vi "internalTesting.vi"() -> ()   [LabVIEW 2017, in "LabVIEW NPOI.lvlib" / "MS-Word.lvclass"]
uses:
  MS-Word.lvclass
  C:/Users/Neo/Desktop/Dev_Tools_BR/LabVIEW_NPOI/src/LabVIEW NPOI/Document/Document.lvclass
  Document/Document.lvclass/Document.ctl
  Document/Set FilePath.vi
panel:
  out "Text 2":string
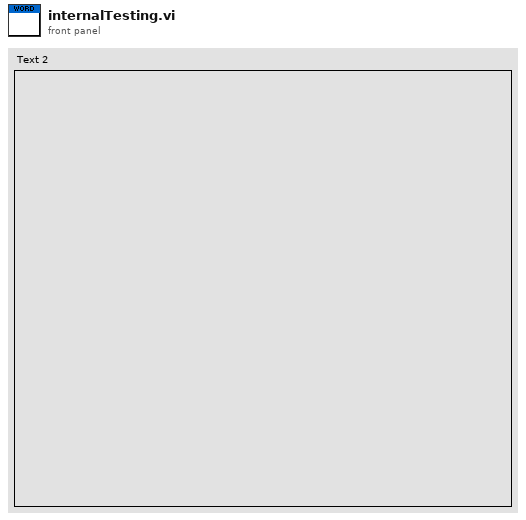
[diagram p1: front panel]
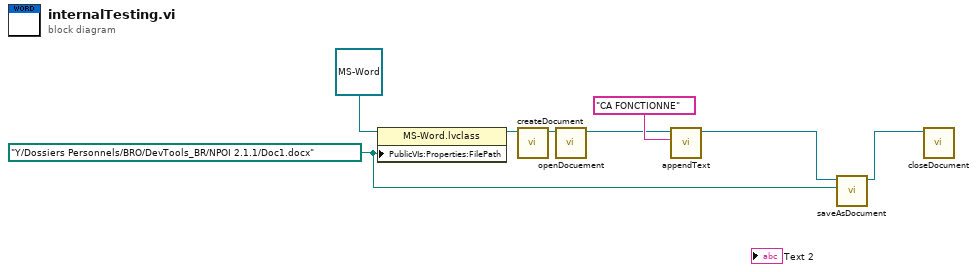
[diagram p0: block diagram]
diagram:
  w6 = path "Y:/Dossiers Personnels/BRO/DevTools_BR/NPOI 2.1.1/Doc1.docx" ("path")
  n1 = property class="MS-Word.lvclass"(reference=refnum<class "MS-Word.lvclass"> refnum ("LabVIEW NPOI.lvlib:MS-Word.lvclass"), "PublicVIs:Properties:FilePath"=w6) -> (reference out=w2:refnum<class "MS-Word.lvclass">)  [unwired: 1 in, 1 out]
  n2 = call-dynamic "createDocument.vi"("MS-Word in"=w2) -> ("MS-Word out"=w1:refnum<class "MS-Word.lvclass">)  [unwired: 9 in, 1 out]
  n3 = call-dynamic "openDocuement.vi"("MS-Word in"=w1) -> ("MS-Word out"=w5:refnum<class "MS-Word.lvclass">)  [unwired: 9 in, 1 out]
  n4 = call-dynamic "appendText.vi"("Text"="CA FONCTIONNE", "MS-Word in"=w5) -> ("MS-Word out"=w4:refnum<class "MS-Word.lvclass">)  [unwired: 8 in, 1 out]
  n5 = call-dynamic "saveAsDocument.vi"("File Path"=w6, "MS-Word in"=w4) -> ("MS-Word out"=w3:refnum<class "MS-Word.lvclass">)  [unwired: 8 in, 1 out]
  n6 = call-dynamic "closeDocument.vi"("MS-Word in"=w3) -> ()  [unwired: 9 in, 2 out]
